vi "TLB Native Dynamic Events ver 0.08a.vi"() -> ()   [LabVIEW 2018]
uses:
  Labview Training Phase 2/Enum Controls/States for Action Engine.ctl
  Type def/TLB event states.ctl
  Type def/TLB MHL States.ctl
  <vilib>/Studica/Studica Toolkit/Background/I2C Channel.ctl
  <vilib>/Studica/Studica Toolkit/NavX/NavX.lvlib
  <vilib>/myRIO/Common/Instrument Driver Framework/myRIO v1.0/AI/typedefs/AI Channels Enum.ctl
  <vilib>/myRIO/Common/Instrument Driver Framework/myRIO v1.0/AI/typedefs/AI Channels List.ctl
  Type def/Type def.ctl
  <vilib>/Studica/Studica Blackhawk/Blackhawk.lvlib
  <vilib>/Studica/Studica Toolkit/Background/Mxp Selection.ctl
  <vilib>/Studica/Studica Toolkit/Background/DIO Channel.ctl
  <vilib>/NI_Real-Time Target Support.lvlib
  <vilib>/ptbypt/NI_PtbyPt.lvlib
  <vilib>/addons/control/pid/NI_PID_pid.lvlib
  Underlying VI's/Webcam FGV Low level ver/State control.ctl
  <vilib>/userdefined/High Color/IMAQdx.ctl
  <vilib>/addons/control/pid/pid.llb/PID (DBL).vi
panel:
  out "Decision":i8
  out "Manual Zero Yaw":bool
  out "Displacement":T1
  out "Fused Heading":dbl
  in  "error in (no error)":errorcluster
  in  "RED LED State":enum16{"OFF", "ON", "BLINK"}(ring)
  in  "GREEN LED State":enum16{"OFF", "ON", "BLINK"}(ring)
  in  "Red LED":bool
  in  "Green LED":bool
  in  "NavX Zero Yaw":bool
  out "Input state":i8
  out "Waveform Chart 2":dbl(graph)
  out "Waveform Chart":dbl(graph)
  in  "STOP":bool
  out "DIO 0":bool
  out "DIO 1":bool
  out "Limit Switch Array":bool[](array[boolean])
  out "error out":errorcluster
  out "L/R average":fxp<+,64,64>
  out "Right Ultrasonic":fxp<+,64,16>
  out "Left Ultrasonic":fxp<+,64,16>
  out "Right IR Sensor":dbl
  out "Left IR Sensor":dbl
  out "Object detection count":T2
  out "Camera error":errorcluster
  in  "Servo Angle":u8(slide) scale=0.0..180.0
  in  "On/Off":bool
  out "Error":errorcluster
  out "element":T3
  out "Action Queue Items":i32
  out "State Logic Queue Items":i32
  out "Action Queues items":string[](array[string])=["Hardware reset", "Software reset", ""]
  out "State logic":T4=enum."Task 2"
  out "Action State":string
  out "Yaw":dbl
  # "TLB FRAMEWORK STATUS"
  # "Camera Status Loop"
  # "Test Programme written by Calvin Loke    Dated: 28 Aug 2019\nTest Programme revised by Dr Alex See   Dated 30 Aug 2019\n\nProgramme version:   TLB Native Dynamic Events ver 0.04b.vi"
  # "Problems now:\nYaw does not work when code is in last state mode\nSlow acceleration due to loop rate?"
  # "Motor Control Loop"
  # "NAVX Control Loop"
  # "Blackhawk status"
  # "Sensor data"
  # "System Health Status Update"
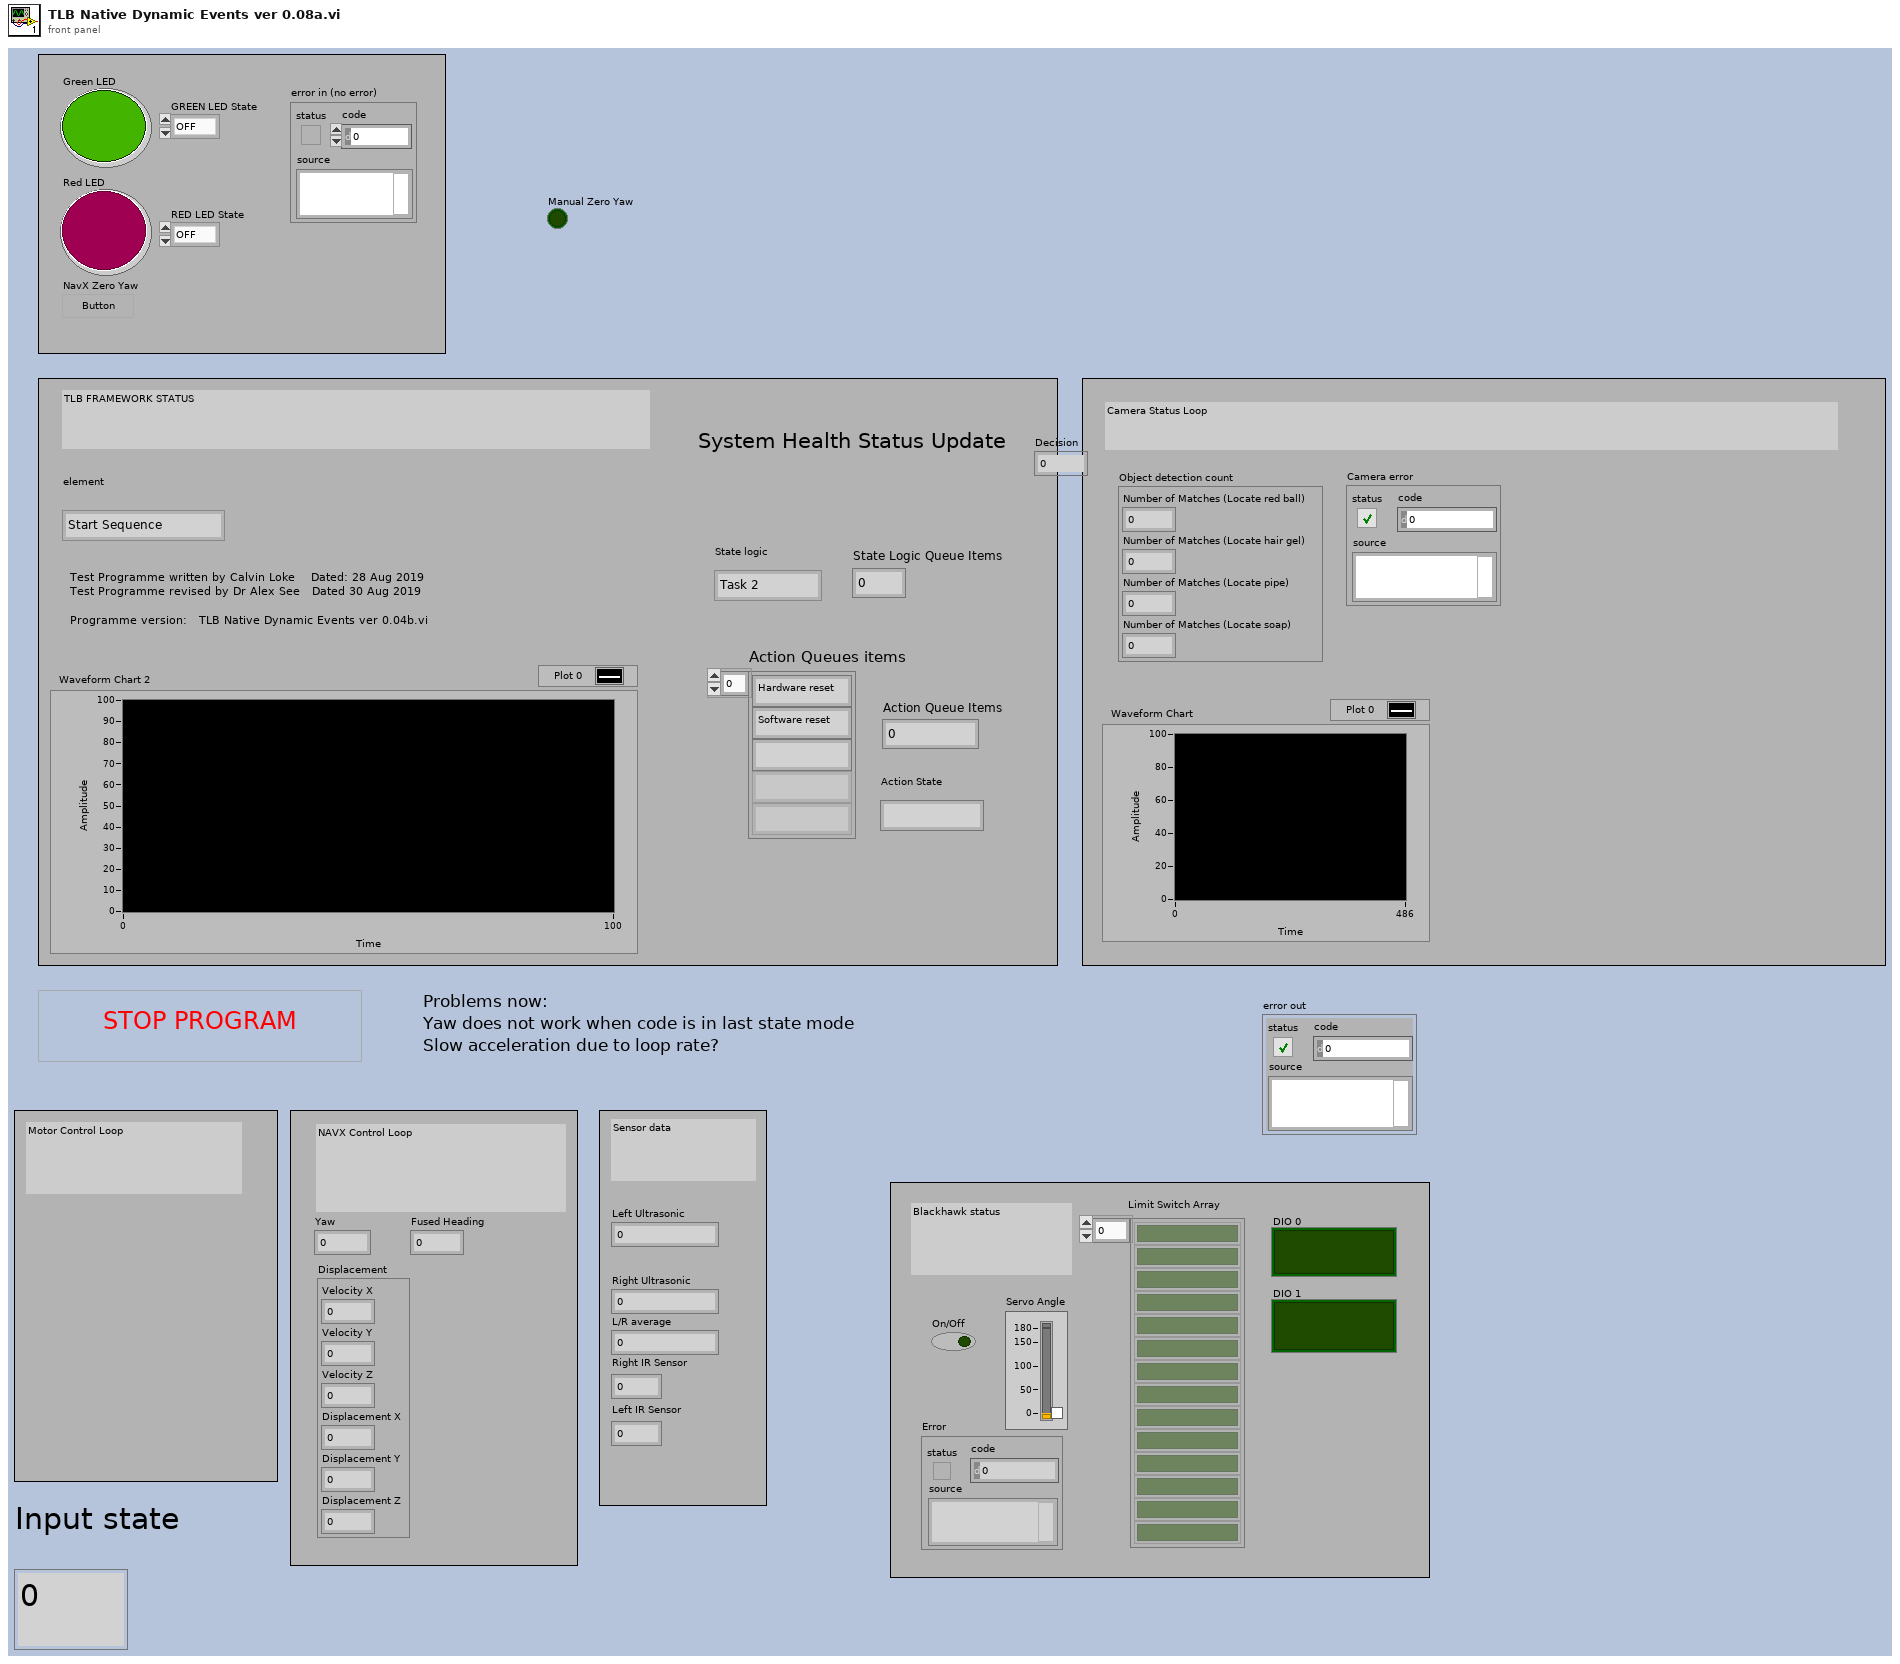
[diagram p1: front panel]
types:
  T1 = cluster{"Velocity X":dbl, "Velocity Y":dbl, "Velocity Z":dbl, "Displacement X":dbl, "Displacement Y":dbl, "Displacement Z":dbl}
  T2 = cluster{"Number of Matches (Locate red ball)":i32, "Number of Matches (Locate hair gel)":i32, "Number of Matches (Locate pipe)":i32, "Number of Matches (Locate soap)":i32}
  T3 = typedef "TLB event states.ctl" = enum16{"Start Sequence", "Exit", "Start Task 1", "Start Task 2", "Start Task 3", "Start Task 4", "Camera vision", "Wall follow mode", "Idle", "Start Drive Straight"}
  T4 = typedef "TLB MHL States.ctl" = enum16{"None", "Startup", "Idle", "Processing", "Shutdown", "Reset", "Task 1", "Task 2", "Task 3", "Task 4", "Task 4a", "Task 4b", "Task 4c", "Task 4d", "Task 4e", "Task 4f", "Task 4g", "Task 4h", "Acquire image", "Wall follow mode", "Autodrive", "Autodrive a"}
  T5 = typedef "States for Action Engine.ctl" = enum16{"Initialize", "Write", "Read"}
  T6 = typedef "DIO Channel.ctl" = enum16{"Not Connected", "A/DIO1", "A/DIO2", "A/DIO3", "A/DIO4", "A/DIO5", "A/DIO6", "A/DIO7", "A/DIO13", "B/DIO1", "B/DIO2", "B/DIO3", "B/DIO4", "B/DIO5", "B/DIO6", "B/DIO7", "B/DIO13", "C/DIO0", "C/DIO1", "C/DIO2", "C/DIO3", "C/DIO4", "C/DIO5", "C/DIO6", "C/DIO7"}
  T7 = typedef "Type def.ctl" = cluster{"Front Ultrasonic Obstruct":bool, "Left Ultrasonic Obstruct":bool, "Right Ultrasonic Obstruct ":bool}
  T8 = typedef "I2C Channel.ctl" = enum16{"Not Connected", "A", "B"}
  T9 = enum16{"LAST STATE", "STOP", "FORWARD", "BACKWARD", "LEFT", "RIGHT", "RCW", "ACW", "INIT", "RESET ENCODERS"}
  T10 = cluster{"proportional gain (Kc)":dbl, "integral time (Ti, min)":dbl, "derivative time (Td, min)":dbl}
  T11 = typedef "State control.ctl" = enum16{"Initialise", "Start camera", "Continuous Acquisition ", "Stop camera", "Dispose all"}
  T12 = typedef "IMAQdx.ctl" = refnum<k21>
  T13 = typedef "Mxp Selection.ctl" = enum16{"MXP A", "MXP B"}
  T14 = enum16{"DISTANCE READ", "STOP", "FORWARD", "BACKWARD", "LEFT", "RIGHT", "RCW", "ACW", "INIT", "RESET ENCODERS"}
  T15 = typedef "AI Channels List.ctl" = T16[]
  T16 = typedef "AI Channels Enum.ctl" = enum16{"Not Connected", "AudioIn/Left", "AudioIn/Right", "C/AI0", "C/AI1", "A/AI0", "A/AI1", "A/AI2", "A/AI3", "A/AI4", "A/AI5", "A/AI6", "A/AI7", "B/AI0", "B/AI1", "B/AI2", "B/AI3", "B/AI4", "B/AI5", "B/AI6", "B/AI7", "AI/AI0", "AI/AI1", "AI/AI2", "AI/AI3", "A/AI0 (DIFF)", "A/AI1 (DIFF)", "A/AI2 (DIFF)", "A/AI3 (DIFF)", "B/AI0 (DIFF)", "B/AI1 (DIFF)", "B/AI2 (DIFF)", "B/AI3 (DIFF)"}
  T17 = cluster{"DIO Channel":T6, "FPGA VI Reference Out":refnum<k20>}
  T18 = typedef "Analog Scaling Constants List.ctl" = T19[]
  T19 = typedef "Analog Scaling Constants.ctl" = cluster{"LSB Weight (Volts)":dbl, "Offset (Volts)":dbl, "Signed?":bool}
  T20 = cluster{"Scale Constants Array":T18, "FPGA Reference Out":refnum<k20>, "AI Channel":T15}
  T21 = cluster{"I2C Channel":T8, "FPGA VI Reference Out":refnum<k20>}
  T22 = typedef "NI_Real-Time Target Support.lvlib/RT CPU Load.ctl" = cluster{"Total (%)":dbl, "Time Critical (%)":dbl, "Timed Structures (%)":dbl, "High (%)":dbl, "Above Normal (%)":dbl, "Normal (%)":dbl, "Background (%)":dbl, "Idle (%)":dbl, "ISR (%)":dbl}
  T23 = cluster{"CPU loads[0]":T22, "CPU loads[1]":T22, "CPU loads[2]":T22, "CPU loads[3]":T22, "CPU loads[4]":T22, "CPU loads[5]":T22, "CPU loads[6]":T22, "CPU loads[7]":T22, "CPU loads[8]":T22}
  T24 = cluster{"I2C Ref Out":cluster{"I2C Channel":T8, "FPGA VI Reference Out":refnum<k20>}, "Connected":bool, "Slave Address (7-bit)":u8, "Registry":u8[]}
  T25 = cluster{"Yaw":dbl, "Roll":dbl, "Pitch":dbl, "Heading":dbl, "Fused Heading":dbl}
  T26 = typedef "IMAQ Image.ctl" = refnum<image>
  T27 = cluster{cluster{"xSpeed":dbl, "ySpeed":dbl, "wSpeed":dbl}, cluster{"xDistance":dbl, "yDistance":dbl, "wDistance":dbl}}
  T28 = cluster{"xDistance":dbl, "yDistance":dbl, "wDistance":dbl}
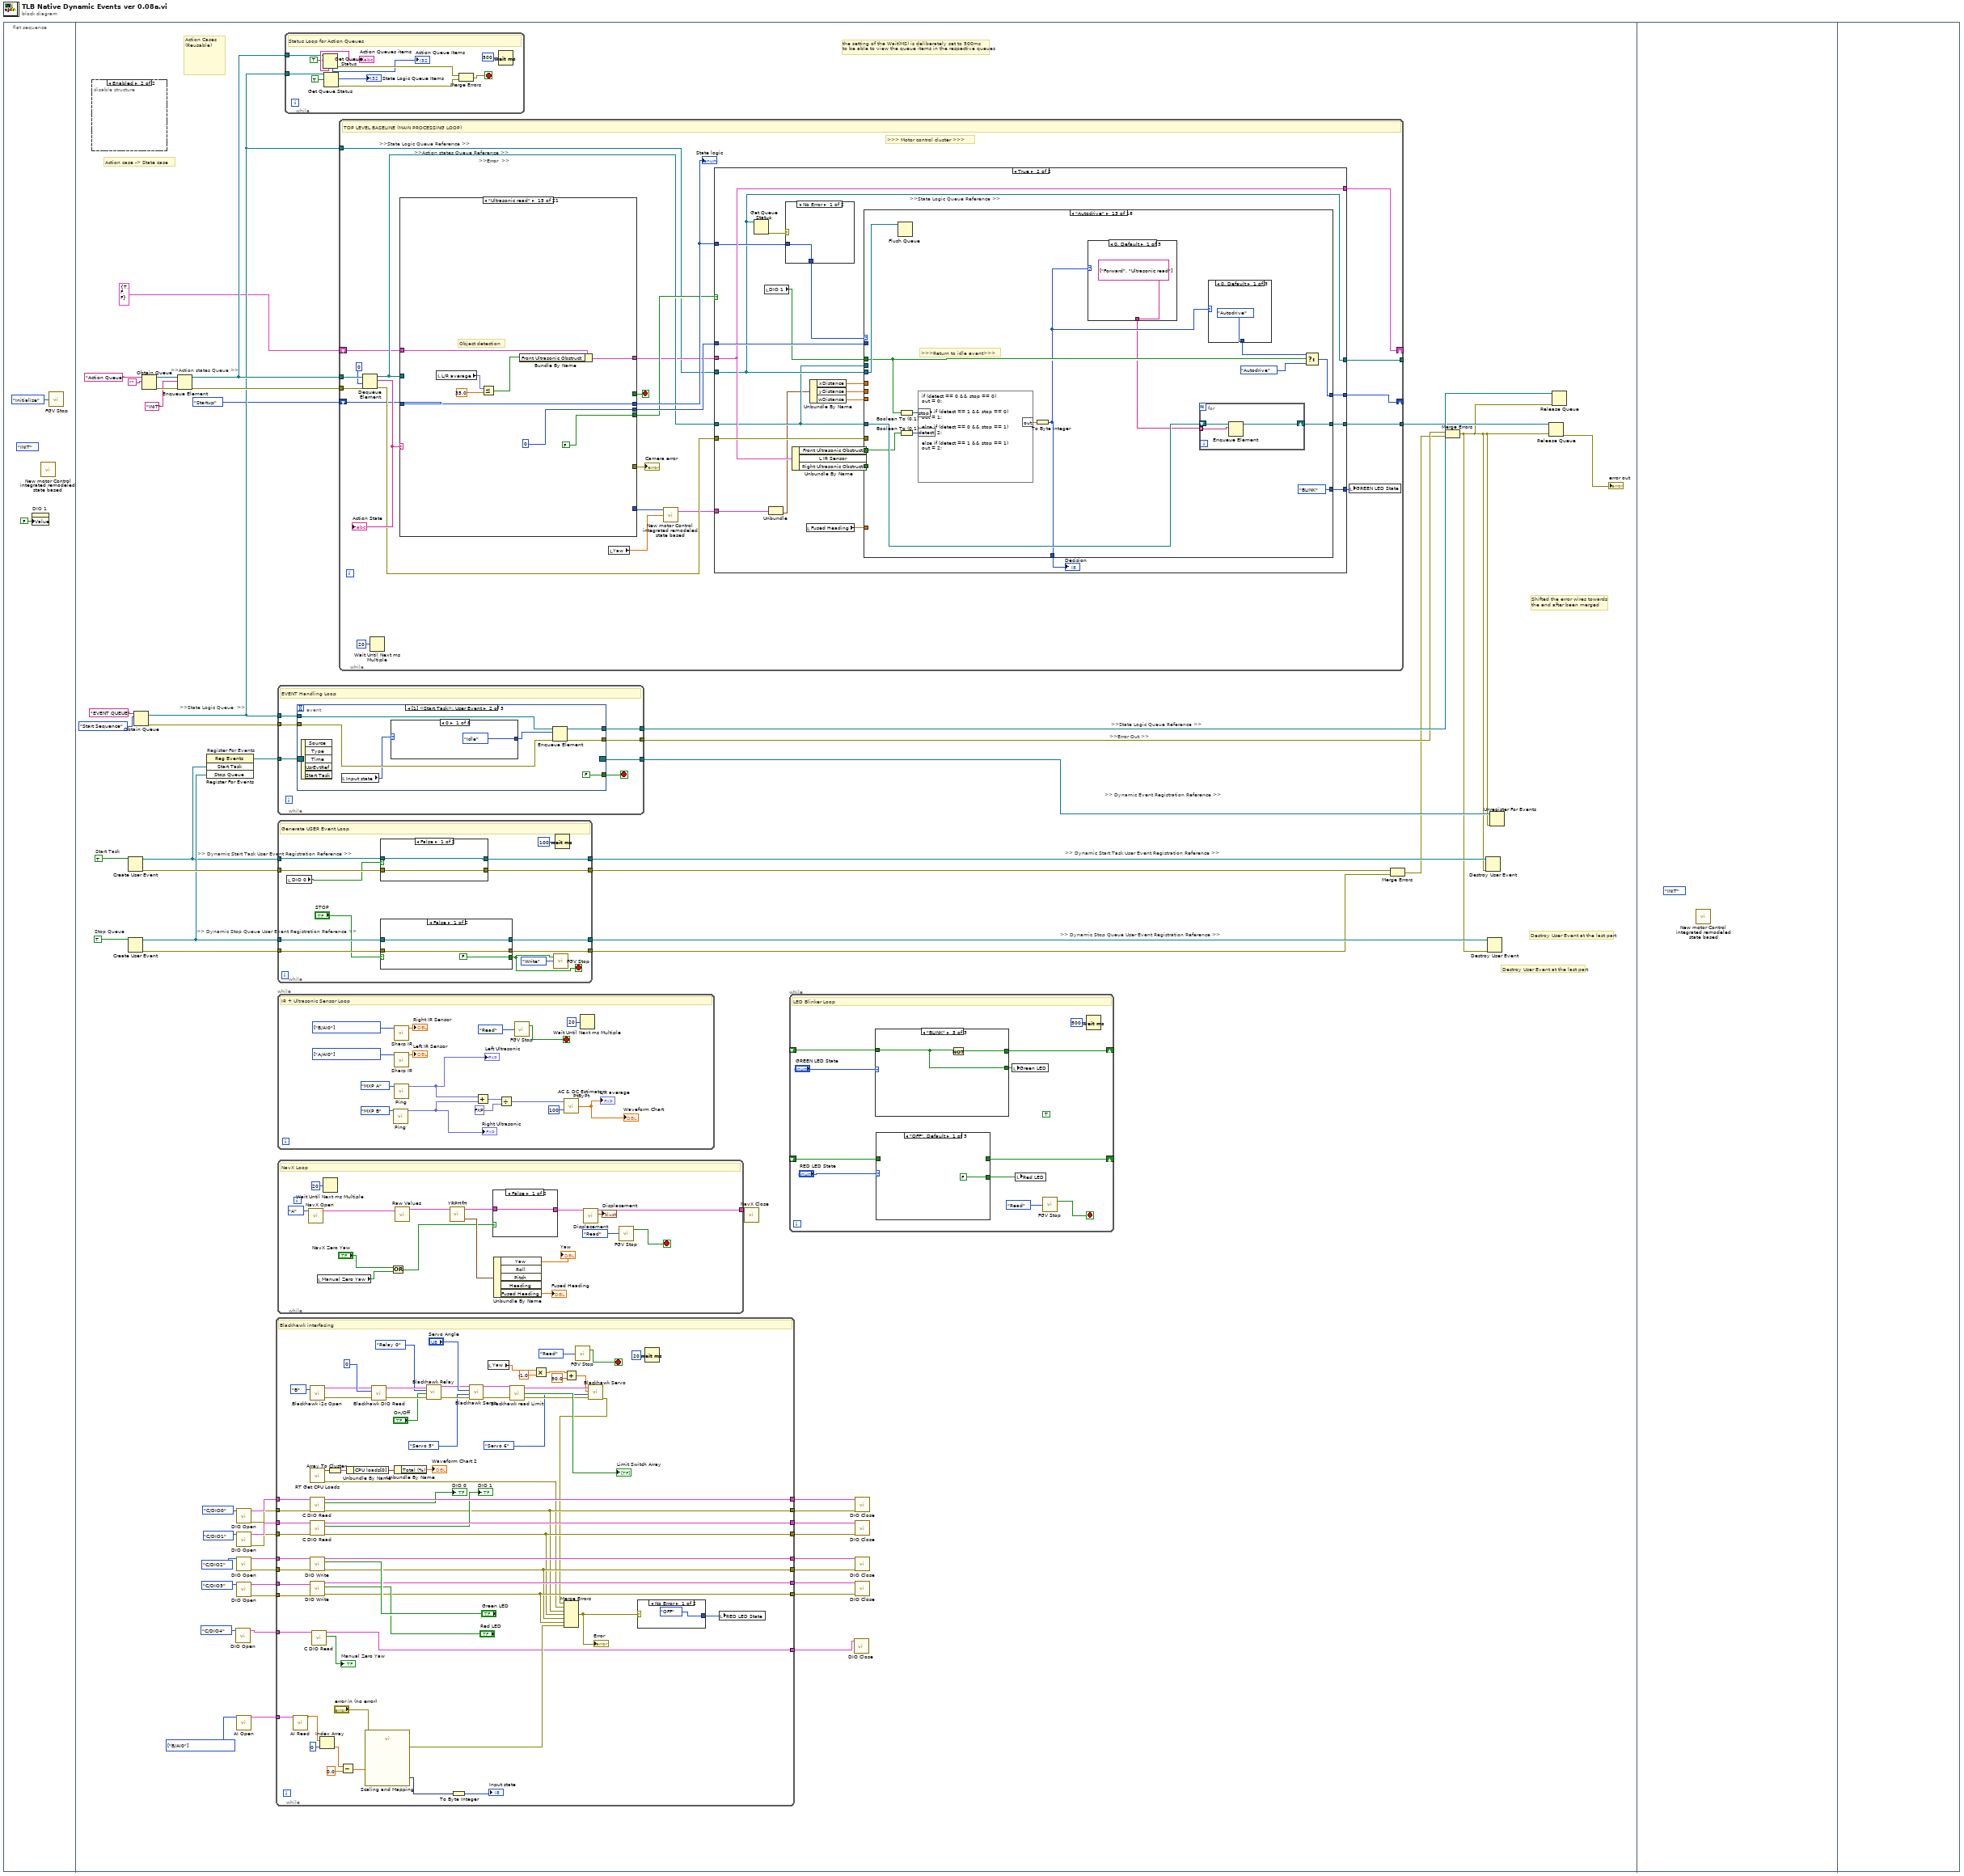
[diagram p0: block diagram]
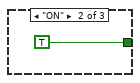
[diagram p2: hidden frame]
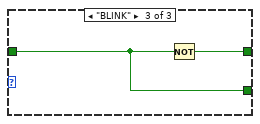
[diagram p3: hidden frame]
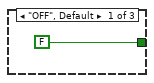
[diagram p4: hidden frame]
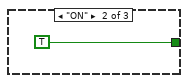
[diagram p5: hidden frame]
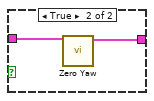
[diagram p6: hidden frame]
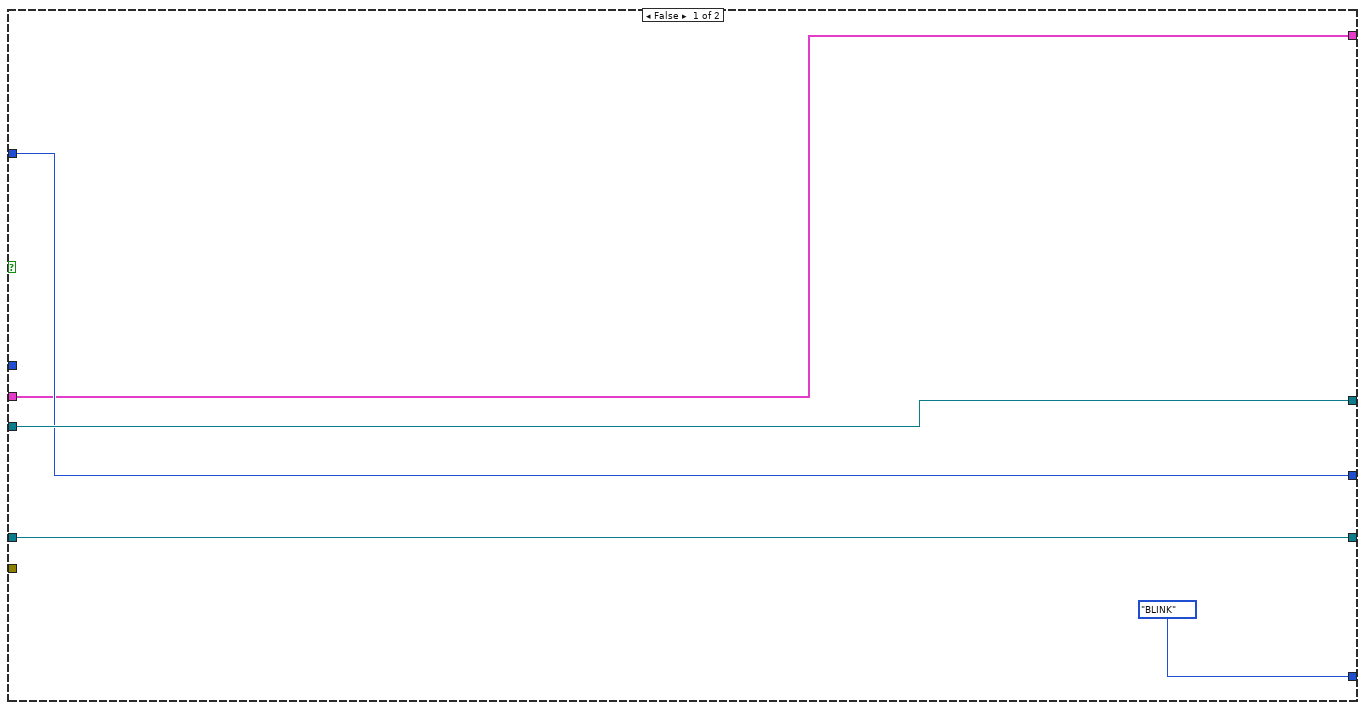
[diagram p7: hidden frame]
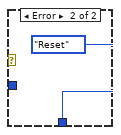
[diagram p8: hidden frame]
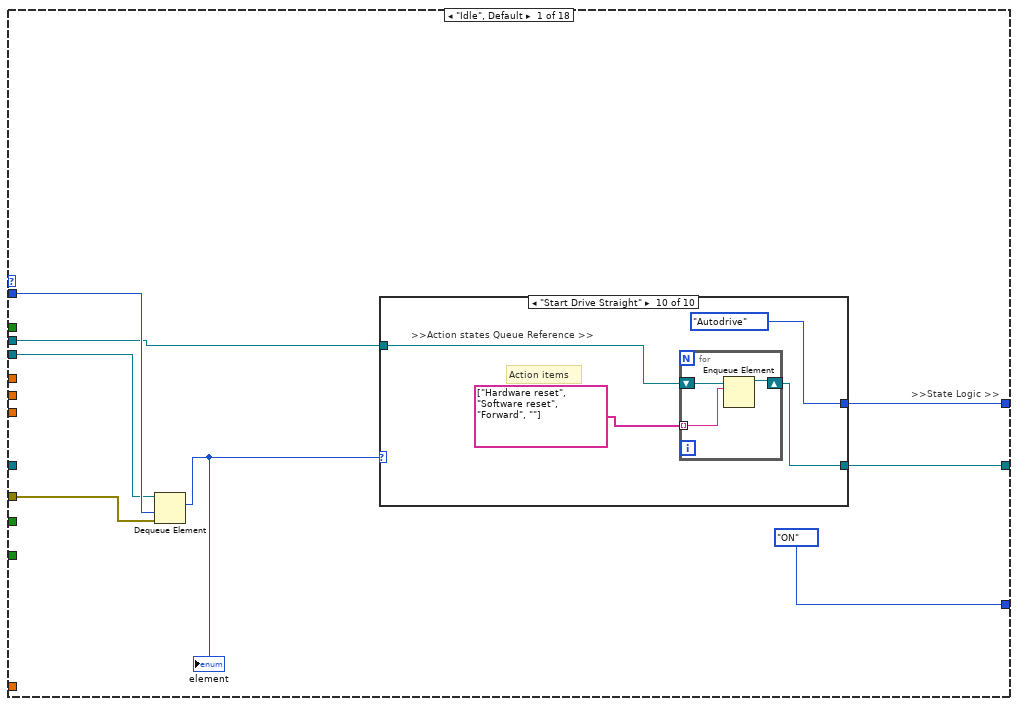
[diagram p9: hidden frame]
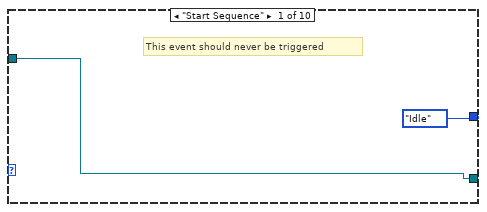
[diagram p10: hidden frame]
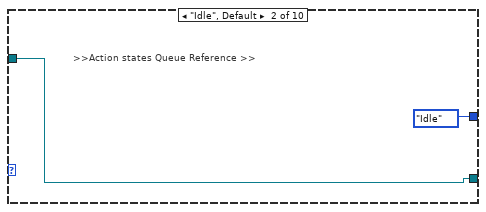
[diagram p11: hidden frame]
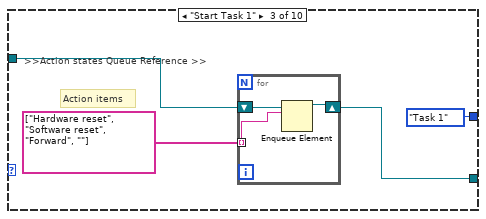
[diagram p12: hidden frame]
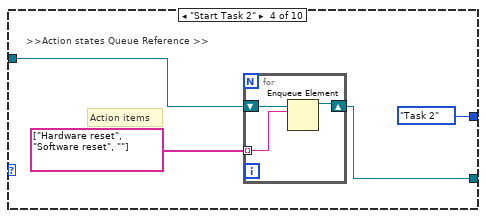
[diagram p13: hidden frame]
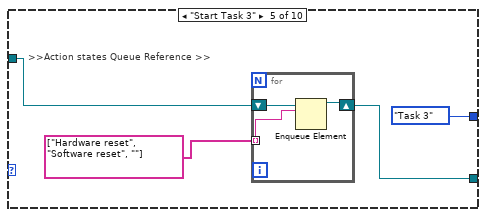
[diagram p14: hidden frame]
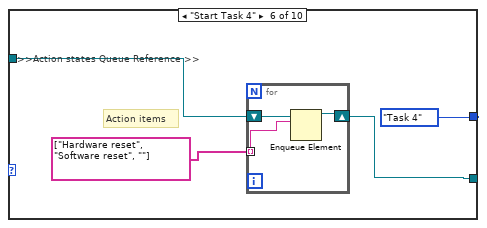
[diagram p15: hidden frame]
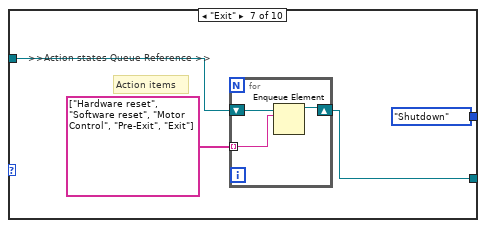
[diagram p16: hidden frame]
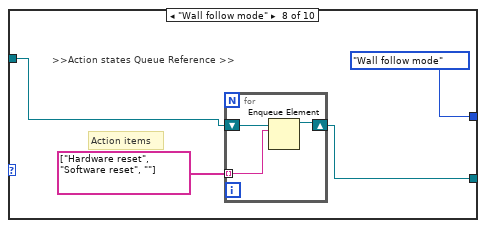
[diagram p17: hidden frame]
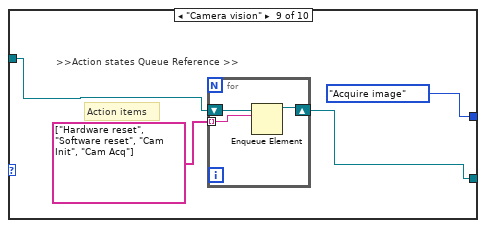
[diagram p18: hidden frame]
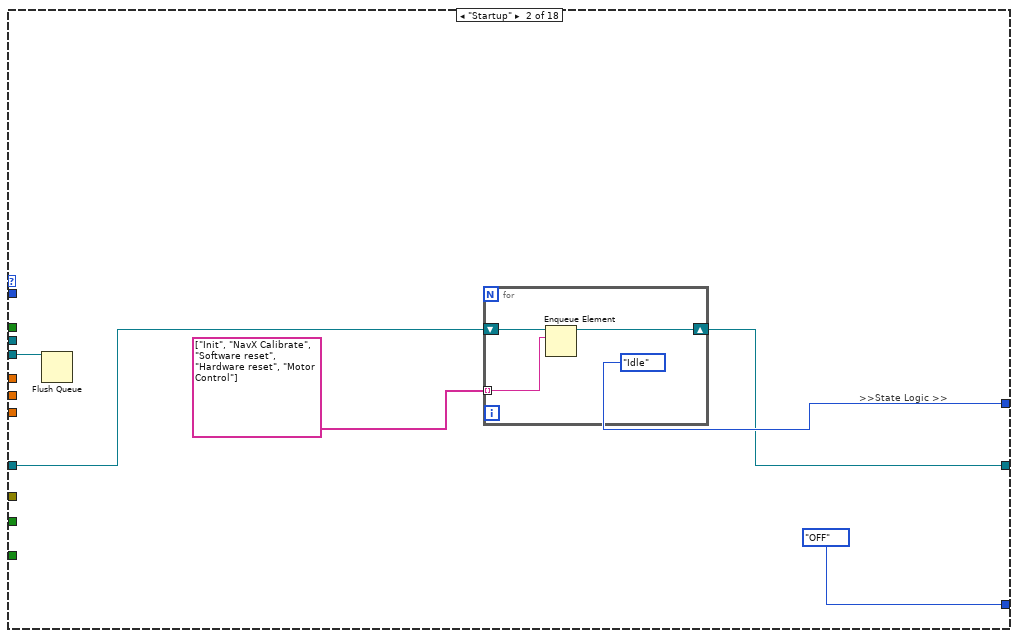
[diagram p19: hidden frame]
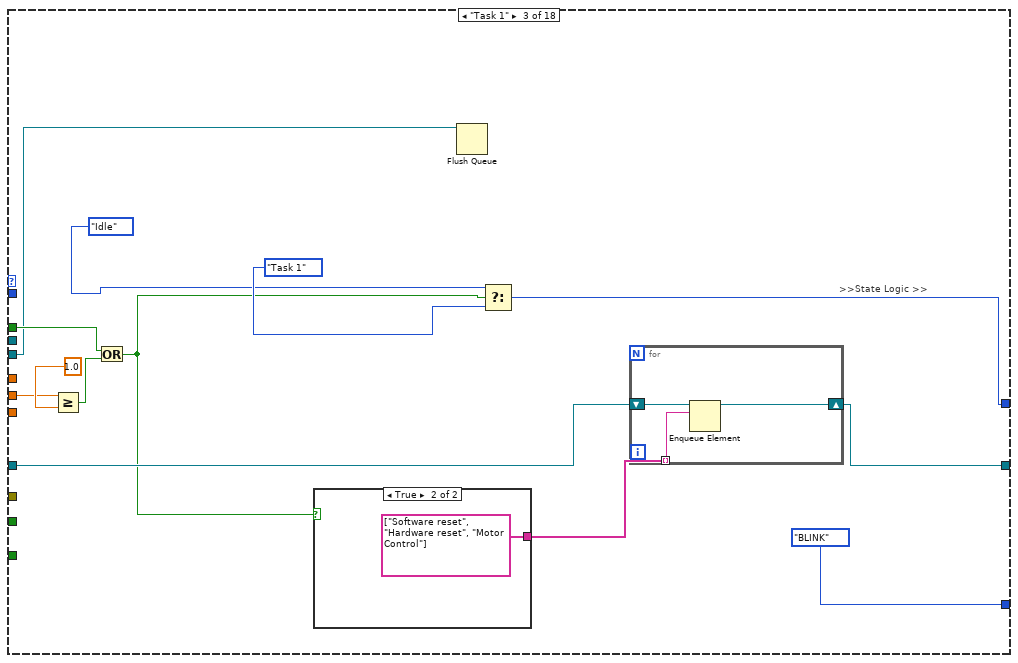
[diagram p20: hidden frame]
diagram:
  n1 = flat-sequence {
    frame #0 {
      (unwired) T14."INIT" ("States")
      n2 = property on="DIO 1" class="Bool (strict)"("Value"=FALSE ("DIO 1")) -> ()  [unwired: 2 in, 2 out]
      n3 = call "New motor Control integrated remodeled state based.vi"() -> ()  [unwired: 3 in, 2 out]
      n4 = call "FGV Stop.vi"("Init/Read/Write State"=States_for_Action_Engine."Initialize") -> ()  [unwired: 2 in, 2 out]
    }
    frame #1 {
      w11 = T15 [enum."B/AI0"] items=["Not Connected", "AudioIn/Left", "AudioIn/Right", "C/AI0", "C/AI1", "A/AI0", "A/AI1", "A/AI2", "A/AI3", "A/AI4", "A/AI5", "A/AI6", "A/AI7", "B/AI0", "B/AI1", "B/AI2", "B/AI3", "B/AI4", "B/AI5", "B/AI6", "B/AI7", "AI/AI0", "AI/AI1", "AI/AI2", "AI/AI3", "A/AI0 (DIFF)", "A/AI1 (DIFF)", "A/AI2 (DIFF)", "A/AI3 (DIFF)", "B/AI0 (DIFF)", "B/AI1 (DIFF)", "B/AI2 (DIFF)", "B/AI3 (DIFF)"] ("AI Channel")
      w59 = TRUE  # Stop Queue
      w58 = TRUE  # Start Task
      # "Action case -> State case"
      # "the setting of the Wait(MS) is deliberately set to 500ms\nto be able to view the queue items in the respective queues"
      # "Action Cases\n(Reusable)"
      # ">>Error Out >>"
      # ">> Dynamic Stop Queue User Event Registration Reference >>"
      # ">> Dynamic Start Task User Event Registration Reference >>"
      # ">> Dynamic Stop Queue User Event Registration Reference >>"
      # ">> Dynamic Start Task User Event Registration Reference >>"
      # ">> Dynamic Event Registration Reference >>"
      # ">>Action states Queue >>"
      # ">>State Logic Queue  >>"
      # ">>State Logic Queue Reference >>"
      # "Destroy User Event at the last part"
      # "Destroy User Event at the last part"
      # "Shifted the error wires towards\nthe end after been merged"
      n5 = disable-structure shown="Enabled" {
        frame Disabled {
          (unwired) variant
          (unwired) TRUE
          n6 = Variant To Data(type="") -> ()  [unwired: 2 in, 2 out]
        }
        frame Enabled {
        }
      }
      n7 = Create User Event(user event datatype=w58) -> (user event=w50:refnum<user-event>, error out=w55:errorcluster)  [unwired: 1 in]
      n8 = Create User Event(user event datatype=w59) -> (user event=w51:refnum<user-event>, error out=w54:errorcluster)  [unwired: 1 in]
      n9 = Obtain Queue(name (unnamed)="EVENT QUEUE", element data type=TLB_event_states."Start Sequence" ("Enum")) -> (queue out=w35:refnum<queue>, error out=w41:errorcluster)  [unwired: 3 in, 1 out]
      n10 = Obtain Queue(name (unnamed)="Action Queue", element data type="") -> (queue out=w44:refnum<queue>, error out=w40:errorcluster)  [unwired: 3 in, 1 out]
      n11 = Enqueue Element(queue=w44, element="INIT", error in (no error)=w40) -> (queue out=w36:refnum<queue>, error out=w39:errorcluster)  [unwired: 1 in, 1 out]
      n12 = register-events "Register For Events"(w50, w51) -> (reference out=w49:refnum<event-registration>)  [unwired: 2 in, 1 out]
      n13 = call <vilib>:"DIO Open.vi"("DIO Channel"=DIO_Channel."C/DIO4") -> ("DIO Info Out"=w5:T17)  [unwired: 9 in, 1 out]
      n14 = call <vilib>:"DIO Open.vi"("DIO Channel"=DIO_Channel."C/DIO0") -> ("error out"=w21:errorcluster, "DIO Info Out"=w27:T17)  [unwired: 9 in]
      n15 = call <vilib>:"DIO Open.vi"("DIO Channel"=DIO_Channel."C/DIO1") -> ("error out"=w19:errorcluster, "DIO Info Out"=w23:T17)  [unwired: 9 in]
      n16 = call <vilib>:"DIO Open.vi"("DIO Channel"=DIO_Channel."C/DIO2") -> ("error out"=w9:errorcluster, "DIO Info Out"=w15:T17)  [unwired: 9 in]
      n17 = call <vilib>:"DIO Open.vi"("DIO Channel"=DIO_Channel."C/DIO3") -> ("error out"=w7:errorcluster, "DIO Info Out"=w14:T17)  [unwired: 9 in]
      n18 = call <vilib>:"AI Open.vi"("AI Channel"=w11) -> ("Analog Info"=w10:T20)  [unwired: 9 in, 1 out]
      n19 = while {
        tunnel: w27 -> [w736]
        tunnel: [w735] -> w26
        tunnel: w23 -> [w734]
        tunnel: [w733] -> w22
        tunnel: w21 -> [w732]
        tunnel: [w701] -> w20
        tunnel: w19 -> [w731]
        tunnel: [w702] -> w18
        tunnel: w15 -> [w725]
        tunnel: w14 -> [w724]
        tunnel: [w721] -> w13
        tunnel: [w720] -> w12
        tunnel: w10 -> [w719]
        tunnel: w9 -> [w712]
        tunnel: [w703] -> w8
        tunnel: w7 -> [w711]
        tunnel: [w704] -> w6
        tunnel: w5 -> [w692]
        tunnel: [w691] -> w3
        stop <- w749 stop-if-true
        # "Blackhawk interfacing"
        n20 = call <vilib>:"AI Read.vi"("Analog Info"=w719) -> ("Array"=w715:dbl[])  [unwired: 9 in, 1 out]
        n21 = call <vilib>:"Blackhawk i2c Open.vi"("I2C Channel"=I2C_Channel."B") -> ("I2C Ref Out"=w727:T21, "error out"=w726:errorcluster)  [unwired: 2 in]
        n22 = call <vilib>:"RT Get CPU Loads.vi"() -> ("error out"=w700:errorcluster, "CPU loads"=w706:T22[])  [unwired: 10 in]
        n23 = call <vilib>:"C DIO Read.vi"("error in (no error)"=w732, "DIO Info In in"=w736) -> ("error out"=w701:errorcluster, "IN"=→"DIO 0":bool, "DIO Info In out"=w735:T17)  [unwired: 7 in]
        n24 = call <vilib>:"C DIO Read.vi"("error in (no error)"=w731, "DIO Info In in"=w734) -> ("error out"=w702:errorcluster, "IN"=→"DIO 1":bool, "DIO Info In out"=w733:T17)  [unwired: 7 in]
        n25 = call <vilib>:"DIO Write.vi"("error in (no error)"=w712, "Input"="Green LED", "DIO Info In"=w725) -> ("error out"=w703:errorcluster, "DIO Info Out"=w721:T17)  [unwired: 7 in]
        n26 = call <vilib>:"DIO Write.vi"("error in (no error)"=w711, "Input"="Red LED", "DIO Info In"=w724) -> ("error out"=w704:errorcluster, "DIO Info Out"=w720:T17)  [unwired: 7 in]
        n27 = call <vilib>:"C DIO Read.vi"("DIO Info In in"=w692) -> ("IN"=→"Manual Zero Yaw":bool, "DIO Info In out"=w691:T17)  [unwired: 8 in, 1 out]
        n28 = Index Array(array=w715, index=0) -> (element=w717:dbl)
        n29 = Array To Cluster(array=w706) -> (cluster=w707:T23)
        n30 = Subtract(x=w717, y=0.0) -> (x-y=w718:dbl)
        n31 = Unbundle By Name(w707) -> ("CPU loads[0]"=w708:T22)
        n32 = call "Scaling and Mapping"("error in (no error)"="error in (no error)", "Signals"=w718) -> ("error out"=w705:errorcluster, "Scaled Signals"=w713:dynamicdata)  [unwired: 8 in]
        n33 = call <vilib>:"Blackhawk DIO Read.vi"("I2C Ref In"=w727, "PIN"=u8 0, "error in (no error)"=w726) -> ("I2C Ref Out"=w747:T21, "error out"=w748:errorcluster)  [unwired: 3 in, 1 out]
        n34 = Unbundle By Name(w708) -> ("Total (%)"=→"Waveform Chart 2":dbl)
        n35 = call <vilib>:"Blackhawk Relay.vi"("error in (no error)"=w748, "On/Off"="On/Off", "Relay"=enum8{"Relay 0", "Relay 1", "Relay 2"}."Relay 0", "I2C Ref In"=w747) -> ("error out"=w744:errorcluster, "I2C Ref Out"=w741:T21)  [unwired: 6 in]
        n36 = To Byte Integer(number=w713) -> (8bit integer=→"Input state":i8)
        n37 = call <vilib>:"Blackhawk Servo.vi"("error in (no error)"=w744, "Servo Select"=enum16{"Servo 5", "Servo 6"}."Servo 5", "Servo Angle"="Servo Angle", "I2C Ref In"=w741) -> ("error out"=w739:errorcluster, "I2C Ref Out"=w738:T21)  [unwired: 6 in]
        n38 = local read "Yaw"() -> (w686:dbl)
        n39 = call <vilib>:"Blackhawk read Limit.vi"("error in (no error)"=w739, "I2C Ref In"=w738) -> ("error out"=w696:errorcluster, "Limit Switch Array"=→"Limit Switch Array":bool[], "I2C Ref Out"=w694:T21)  [unwired: 1 in]
        n40 = Multiply(x=w686, y=-1.0) -> (x*y=w687:dbl)
        n41 = Add(x=w687, y=90.0) -> (x+y=w688:dbl)
        n42 = call "FGV Stop.vi"("Init/Read/Write State"=States_for_Action_Engine."Read") -> ("Output node"=w749:bool)  [unwired: 2 in, 1 out]
        n43 = call <vilib>:"Blackhawk Servo.vi"("error in (no error)"=w696, "Servo Select"=enum16{"Servo 5", "Servo 6"}."Servo 6", "Servo Angle"=w688, "I2C Ref In"=w694) -> ("error out"=w695:errorcluster)  [unwired: 6 in, 1 out]
        n44 = Merge Errors(w695, w700, w701, w702, w703, w704, w705) -> (w699:errorcluster)
        "Error" <- w699
        n45 = case shown="No Error" w699 {
          tunnel: [enum16{"OFF", "ON", "BLINK"}."OFF" ("RED LED State") enum16{"OFF", "ON", "BLINK"}."BLINK" ("RED LED State")] -> w710
          frame No Error {
          }
          frame Error {
          }
        }
        n46 = Wait (ms)(milliseconds to wait=u32 20) -> ()  [unwired: 1 out]
        n47 = local write "RED LED State"(w710) -> ()
      }
      n48 = while {
        tunnel: w49 -> [w629]
        tunnel: [w628] -> w48
        tunnel: w35 -> [w626]
        tunnel: [w625] -> w47
        tunnel: w41 -> [w624]
        tunnel: [w623] -> w38
        stop <- w627 stop-if-true
        # "EVENT Handling Loop"
        n49 = event shown="[1] <Start Task>: User Event" {
          selector: w629 -> [_ _ _]
          dyn-events: [_ _ _] -> w628
          timeout: _ -> [_ _ _]
          tunnel: [FALSE FALSE w656] -> w627
          tunnel: w626 -> [w634 w641 w654]
          tunnel: [w633 w640 w655] -> w625
          tunnel: w624 -> [w631 w639 w652]
          tunnel: [w630 w638 w651] -> w623
          event Timeout {
            n50 = event-data() -> ()  [unwired: 1 in, 3 out]
            n51 = Enqueue Element(queue=w634, element=TLB_event_states."Idle" ("Enum"), error in (no error)=w631) -> (queue out=w633:refnum<queue>, error out=w630:errorcluster)  [unwired: 1 in, 1 out]
          }
          event User Event {
            n52 = event-data() -> ()  [unwired: 1 in, 5 out]
            n53 = local read "Input state"() -> (w637:i8)
            n54 = case shown="0" w637 {
              tunnel: [TLB_event_states."Idle" ("Enum") TLB_event_states."Start Task 1" ("Enum") TLB_event_states."Start Task 2" ("Enum") TLB_event_states."Start Task 3" ("Enum") TLB_event_states."Start Task 4" ("Enum") TLB_event_states."Wall follow mode" ("Enum") TLB_event_states."Camera vision" ("Enum") TLB_event_states."Start Drive Straight" ("Enum")] -> w636
              frame 0 {
              }
              frame 1 {
              }
              frame 2 {
              }
              frame 3, Default {
              }
              frame 4 {
              }
              frame 5 {
              }
              frame 6 {
              }
              frame 7 {
              }
            }
            n55 = Enqueue Element(queue=w641, element=w636, error in (no error)=w639) -> (queue out=w640:refnum<queue>, error out=w638:errorcluster)  [unwired: 1 in, 1 out]
          }
          event User Event {
            n56 = event-data() -> ("Stop Queue"=w656:bool)  [unwired: 1 in, 4 out]
            n57 = Enqueue Element At Opposite End(queue=w654, element=TLB_event_states."Exit" ("Enum"), error in (no error)=w652) -> (queue out=w655:refnum<queue>, error out=w651:errorcluster)  [unwired: 1 in, 1 out]
          }
        }
      }
      n58 = while {
        tunnel: w50 -> [w668]
        tunnel: w51 -> [w667]
        tunnel: [w666] -> w57
        tunnel: [w665] -> w56
        tunnel: w55 -> [w664]
        tunnel: [w663] -> w53
        tunnel: w54 -> [w662]
        tunnel: [w661] -> w52
        stop <- w659 stop-if-true
        # "Generate USER Event Loop"
        n59 = local read "DIO 0"() -> (w658:bool)
        n60 = case shown="False" w658 {
          selector: w658 -> [_ w680]
          tunnel: w668 -> [w679 w684]
          tunnel: [w679 w683] -> w665
          tunnel: w664 -> [w678 w682]
          tunnel: [w678 w681] -> w663
          frame False {
          }
          frame True {
            n61 = Generate User Event(user event=w684, event data cluster=w680, error in=w682) -> (user event out=w683:refnum<user-event>, error out=w681:errorcluster)  [unwired: 1 in]
          }
        }
        n62 = case shown="False" "STOP" {
          selector: "STOP" -> [_ w673]
          tunnel: w667 -> [w672 w677]
          tunnel: [w672 w676] -> w666
          tunnel: w662 -> [w671 w675]
          tunnel: [w671 w674] -> w661
          tunnel: [FALSE w673] -> w659
          frame False {
          }
          frame True {
            n63 = Generate User Event(user event=w677, event data cluster=w673, error in=w675) -> (user event out=w676:refnum<user-event>, error out=w674:errorcluster)  [unwired: 1 in]
          }
        }
        n64 = call "FGV Stop.vi"("Init/Read/Write State"=States_for_Action_Engine."Write", "Input Node"=w659) -> ()  [unwired: 1 in, 2 out]
        n65 = Wait (ms)(milliseconds to wait=u32 100) -> ()  [unwired: 1 out]
      }
      n66 = while {
        stop <- w605 stop-if-true
        w610 = T15 [enum."A/AI0"] items=["Not Connected", "AudioIn/Left", "AudioIn/Right", "C/AI0", "C/AI1", "A/AI0", "A/AI1", "A/AI2", "A/AI3", "A/AI4", "A/AI5", "A/AI6", "A/AI7", "B/AI0", "B/AI1", "B/AI2", "B/AI3", "B/AI4", "B/AI5", "B/AI6", "B/AI7", "AI/AI0", "AI/AI1", "AI/AI2", "AI/AI3", "A/AI0 (DIFF)", "A/AI1 (DIFF)", "A/AI2 (DIFF)", "A/AI3 (DIFF)", "B/AI0 (DIFF)", "B/AI1 (DIFF)", "B/AI2 (DIFF)", "B/AI3 (DIFF)"] ("AI Channel")
        w611 = T15 [enum."B/AI0"] items=["Not Connected", "AudioIn/Left", "AudioIn/Right", "C/AI0", "C/AI1", "A/AI0", "A/AI1", "A/AI2", "A/AI3", "A/AI4", "A/AI5", "A/AI6", "A/AI7", "B/AI0", "B/AI1", "B/AI2", "B/AI3", "B/AI4", "B/AI5", "B/AI6", "B/AI7", "AI/AI0", "AI/AI1", "AI/AI2", "AI/AI3", "A/AI0 (DIFF)", "A/AI1 (DIFF)", "A/AI2 (DIFF)", "A/AI3 (DIFF)", "B/AI0 (DIFF)", "B/AI1 (DIFF)", "B/AI2 (DIFF)", "B/AI3 (DIFF)"] ("AI Channel")
        # "IR + Ultrasonic Sensor Loop"
        n67 = call <vilib>:"Ping.vi"("Mxp Side"=Mxp_Selection."MXP B") -> ("CM"=w599:fxp<+,64,16>)  [unwired: 8 in, 2 out]
        "Right Ultrasonic" <- w599
        n68 = call <vilib>:"Ping.vi"("Mxp Side"=Mxp_Selection."MXP A") -> ("CM"=w600:fxp<+,64,16>)  [unwired: 8 in, 2 out]
        "Left Ultrasonic" <- w600
        n69 = call <vilib>:"Sharp IR.vi"("AI Channel"=w611) -> ("Sharp IR Distance"=→"Right IR Sensor":dbl)  [unwired: 8 in, 2 out]
        n70 = call <vilib>:"Sharp IR.vi"("AI Channel"=w610) -> ("Sharp IR Distance"=→"Left IR Sensor":dbl)  [unwired: 8 in, 2 out]
        n71 = Add(x=w600, y=w599) -> (x+y=w602:fxp<+,64,17>)
        n72 = Divide(x=w602, y=fxp<+,64,17> 2.0) -> (x/y=w598:fxp<+,64,64>)
        n73 = call "FGV Stop.vi"("Init/Read/Write State"=States_for_Action_Engine."Read") -> ("Output node"=w605:bool)  [unwired: 2 in, 1 out]
        n74 = call <vilib>:"AC & DC Estimator PtByPt.vi"("signal"=w598, "sample length"=100) -> ("DC estimate (V)"=→"L/R average" →"Waveform Chart":dbl)  [unwired: 1 in, 2 out]
        n75 = Wait Until Next ms Multiple(millisecond multiple=u32 20) -> ()  [unwired: 1 out]
      }
      n76 = while {
        tunnel: [w85] -> w28
        stop <- w93 stop-if-true
        # "NavX Loop"
        n77 = call <vilib>:"NavX Open.vi"("I2C Channel"=I2C_Channel."A") -> ("NavX Info"=w87:T24)  [unwired: 9 in, 1 out]
        n78 = local read "Manual Zero Yaw"() -> (w81:bool)
        n79 = Wait Until Next ms Multiple(millisecond multiple=u32 20) -> ()  [unwired: 1 out]
        n80 = Or(x="NavX Zero Yaw", y=w81) -> (x .or. y?=w82:bool)
        n81 = call <vilib>:"Raw Values.vi"("NavX Info In"=w87) -> ("NavX Info Out"=w90:T24)  [unwired: 8 in, 1 out]
        n82 = call <vilib>:"YRPHfH.vi"("NavX Info In"=w90) -> ("YRPHfH"=w91:T25, "NavX Info Out"=w89:T24)  [unwired: 3 in]
        n83 = case shown="False" w82 {
          tunnel: [w95 w97] -> w86
          tunnel: w89 -> [w95 w96]
          frame False {
          }
          frame True {
            n84 = call <vilib>:"Zero Yaw.vi"("NavX Info In"=w96) -> ("NavX Info Out"=w97:T24)  [unwired: 10 in]
          }
        }
        n85 = Unbundle By Name(w91) -> ("Yaw"=→"Yaw":dbl, "Fused Heading"=→"Fused Heading":dbl)  [unwired: 3 out]
        n86 = call <vilib>:"Displacement.vi"("NavX Info In"=w86) -> ("Displacement"=→"Displacement":T1, "NavX Info Out"=w85:T24)  [unwired: 9 in]
        n87 = call "FGV Stop.vi"("Init/Read/Write State"=States_for_Action_Engine."Read") -> ("Output node"=w93:bool)  [unwired: 2 in, 1 out]
      }
      n88 = while {
        tunnel: w36 -> [w620]
        tunnel: w35 -> [w617]
        stop <- w614 stop-if-true
        # "Status Loop for Action Queues"
        n89 = Get Queue Status(queue=w620, return elements? (F)=TRUE) -> (error out=w616:errorcluster, # elements in queue=→"Action Queue Items":i32, elements=→"Action Queues items":string[])  [unwired: 1 in, 5 out]
        n90 = Get Queue Status(queue=w617, return elements? (F)=TRUE) -> (# pending remove=→"State Logic Queue Items":i32, error out=w615:errorcluster)  [unwired: 1 in, 6 out]
        n91 = Merge Errors(w616, w615) -> (w614:errorcluster)
        n92 = Wait (ms)(milliseconds to wait=u32 500) -> ()  [unwired: 1 out]
      }
      n93 = while {
        tunnel: w35 -> [w104]
        shift-right: [w115] -> _
        shift-left: TLB_MHL_States."Startup" ("Enum") -> [w109]
        tunnel: w36 -> [w120]
        tunnel: w39 -> [w118]
        tunnel: [w117] -> _
        tunnel: [w116] -> w31
        shift-right: [w106] -> _
        shift-left: T7 {"Front Ultrasonic Obstruct"=TRUE, "Left Ultrasonic Obstruct"=FALSE, "Right Ultrasonic Obstruct "=FALSE} -> [w108]
        stop <- w102 stop-if-true
        # ">>> Motor control cluster >>>"
        # ">>Error  >>"
        # ">>Action states Queue Reference >>"
        # ">>State Logic Queue Reference >>"
        # "TOP LEVEL BASELINE (MAIN PROCESSING LOOP)"
        n94 = Dequeue Element(queue=w120, timeout in ms (-1)=0, error in (no error)=w118) -> (queue out=w110:refnum<queue>, element=w119:string, error out=w111:errorcluster)  [unwired: 1 out]
        "Action State" <- w119
        n95 = Wait Until Next ms Multiple(millisecond multiple=u32 20) -> ()  [unwired: 1 out]
        n96 = case shown="\"Ultrasonic read\"" w119 {
          tunnel: [w446 w461 w468 w473 w479 w486 w492 w496 w504 w509 w518 w525 TLB_MHL_States."Shutdown" ("Enum") w535 w544 w547 w558 w569 w577 w589 w593] -> w121
          tunnel: [w449 0 0 0 0 0 0 0 0 0 0 0 0 0 0 0 0 0 0 0 0] -> w114
          tunnel: [TRUE FALSE FALSE FALSE FALSE FALSE FALSE FALSE FALSE FALSE FALSE FALSE FALSE FALSE FALSE FALSE FALSE FALSE FALSE FALSE FALSE] -> w113
          tunnel: w110 -> [_ _ _ _ _ _ _ _ _ _ _ _ _ _ _ _ _ _ _ _ _]
          tunnel: w109 -> [w446 w461 w468 w473 w479 w486 w492 w496 w504 w509 w518 w525 _ w535 w544 w547 w558 w569 w577 w589 w593]
          tunnel: w108 -> [w447 w456 w464 w474 w476 w482 w488 w494 w500 w506 w515 w521 w528 w536 w543 w550 w559 w570 w576 w586 w594]
          tunnel: [w447 w455 w463 w474 w476 w482 w488 w494 w500 w506 w514 w521 w528 w536 w540 w549 w559 w570 w576 w586 w594] -> w107
          tunnel: [_ _ _ _ _ _ _ _ _ _ _ _ _ _ _ _ _ w560 w572 w580 _] -> w105
          tunnel: [_ _ _ _ _ _ _ _ _ _ _ _ TRUE _ _ _ _ _ _ _ _] -> w102
          tunnel: [T9."LAST STATE" ("Move mode") T9."INIT" ("Move mode") T9."FORWARD" ("Move mode") T9."LAST STATE" ("Move mode") T9."BACKWARD" ("Move mode") T9."RIGHT" ("Move mode") T9."LEFT" ("Move mode") T9."RCW" ("Move mode") T9."ACW" ("Move mode") T9."STOP" ("Move mode") _ T9."RESET ENCODERS" ("Move mode") T9."INIT" ("Move mode") T9."INIT" ("Move mode") _ _ _ _ _ _ _] -> w100
          frame "No action", Default {
            n97 = case shown="\"Startup\", Default" w446 {
              tunnel: [0 100] -> w449
              frame "Startup", Default {
              }
              frame "Idle" {
              }
            }
            n98 = local write "NavX Zero Yaw"(FALSE ("NavX Zero Yaw")) -> ()
          }
          frame "Init" {
            # ">>State Logic  >>"
            n99 = local write "Servo Angle"(u8 90 ("Servo Angle")) -> ()
            n100 = Bundle By Name(cluster=w456, "Front Ultrasonic Obstruct"=FALSE ("Object detected"), "L IR Sensor"=0.0, "Right Ultrasonic Obstruct"=FALSE ("In move state?")) -> (w455:T7)
          }
          frame "Forward" {
            n101 = local write "NavX Zero Yaw"(FALSE ("NavX Zero Yaw")) -> ()
            n102 = Bundle By Name(cluster=w464, "Right Ultrasonic Obstruct"=TRUE ("In move state?")) -> (w463:T7)
          }
          frame " Motor Control" {
          }
          frame "Reverse" {
            n103 = local write "NavX Zero Yaw"(FALSE ("NavX Zero Yaw")) -> ()
          }
          frame "Right" {
            n104 = local write "NavX Zero Yaw"(FALSE ("NavX Zero Yaw")) -> ()
          }
          frame "Left" {
            n105 = local write "NavX Zero Yaw"(FALSE ("NavX Zero Yaw")) -> ()
          }
          frame "Rotate CW" {
            n106 = local write "NavX Zero Yaw"(FALSE ("NavX Zero Yaw")) -> ()
          }
          frame "Rotate ACW" {
            n107 = local write "NavX Zero Yaw"(FALSE ("NavX Zero Yaw")) -> ()
          }
          frame "Stop" {
            n108 = local write "NavX Zero Yaw"(FALSE ("NavX Zero Yaw")) -> ()
          }
          frame "Software reset" {
            w511 = FALSE ("NavX Zero Yaw")
            n109 = Wait (ms)(milliseconds to wait=u32 20) -> ()  [unwired: 1 out]
            n110 = local write "NavX Zero Yaw"(w511) -> ()
            n111 = Bundle By Name(cluster=w515, "Front Ultrasonic Obstruct"=w511, "L IR Sensor"=0.0, "Right Ultrasonic Obstruct"=w511) -> (w514:T7)
          }
          frame "Hardware reset" {
            n112 = Wait (ms)(milliseconds to wait=u32 100) -> ()  [unwired: 1 out]
            n113 = local write "NavX Zero Yaw"(TRUE ("NavX Zero Yaw")) -> ()
          }
          frame "Exit" {
          }
          frame "Pre-Exit" {
          }
          frame "Ultrasonic read" {
            # "Object detection"
            n114 = local read "L/R average"() -> (w537:fxp<+,64,64>)
            n115 = Less Or Equal?(x=w537, y=35.0) -> (x <= y?=w538:bool)
            n116 = Bundle By Name(cluster=w543, "Front Ultrasonic Obstruct"=w538) -> (w540:T7)
          }
          frame "IR Sensor Read" {
            n117 = local read "Left IR Sensor"() -> (w548:dbl)
            n118 = Bundle By Name(cluster=w550, "L IR Sensor"=w548) -> (w549:T7)
          }
          frame "Calculate" {
            n119 = Unbundle By Name(w559) -> ("L IR Sensor"=w554:dbl)
            n120 = call-poly <vilib>:"PID.vi"("output range"=cluster{"output high":dbl, "output low":dbl} {"output high"=0.3, "output low"=-0.3}, "PID gains"=T10 {"proportional gain (Kc)"=0.01, "integral time (Ti, min)"=0.0, "derivative time (Td, min)"=0.0}, "process variable"=w554, "setpoint"=20.0) -> ("output"=w551:dbl)  [unwired: 6 in, 1 out]
            n121 = Negate(x=w551) -> ()  [unwired: 1 out]
          }
          frame "Cam Init" {
            n122 = call "Low-Level Grab.vi"("States"=State_control."Initialise", "Session In"=T12 "cam1") -> ("error out"=w561:errorcluster, "Session Out"=w562:T12)  [unwired: 7 in, 1 out]
            n123 = call "Low-Level Grab.vi"("error in (no error)"=w561, "States"=State_control."Start camera", "Session In"=w562) -> ("error out"=w560:errorcluster)  [unwired: 6 in, 2 out]
            n124 = local write "Servo Angle"(u8 170 ("Servo Angle")) -> ()
          }
          frame "Cam Acq" {
            n125 = call "Low-Level Grab.vi"("States"=State_control."Continuous Acquisition ") -> ("error out"=w573:errorcluster, "Image Out"=w574:T26)  [unwired: 8 in, 1 out]
            n126 = call "All object detection ver2.vi"("Image In"=w574, "error in"=w573) -> ("Object detection count"=→"Object detection count":T2, "error out"=w572:errorcluster)  [unwired: 1 out]
          }
          frame "Cam Exit" {
            n127 = call "Low-Level Grab.vi"("States"=State_control."Stop camera") -> ("error out"=w581:errorcluster, "Session Out"=w583:T12)  [unwired: 8 in, 1 out]
            n128 = local write "Servo Angle"(u8 90 ("Servo Angle")) -> ()
            n129 = call "Low-Level Grab.vi"("error in (no error)"=w581, "States"=State_control."Dispose all", "Session In"=w583) -> ("error out"=w580:errorcluster)  [unwired: 6 in, 2 out]
          }
          frame "NavX Calibrate" {
            # "Adds a 15 second delay to the startup process \nfor the NavX to calibrate"
            n130 = Wait (ms)(milliseconds to wait=u32 15000) -> ()  [unwired: 1 out]
          }
        }
        "State logic" <- w121
        "Camera error" <- w105
        n131 = local read "Yaw"() -> (w98:dbl)
        n132 = call "New motor Control integrated remodeled state based.vi"("Yaw"=w98, "States"=w100) -> ("Speed and distance cluster"=w99:T27)  [unwired: 1 in, 1 out]
        n133 = case shown="True" w113 {
          tunnel: w121 -> [w125 w136]
          tunnel: w104 -> [w126 w135]
          tunnel: w110 -> [w124 w131]
          tunnel: [w126 w135] -> w117
          tunnel: [w124 w147] -> w116
          tunnel: [w125 w146] -> w115
          tunnel: w111 -> [_ w145]
          tunnel: w114 -> [_ w144]
          tunnel: w107 -> [w123 w138]
          tunnel: [w123 w138] -> w106
          tunnel: [enum16{"OFF", "ON", "BLINK"}."BLINK" ("GREEN LED State") w132] -> w101
          tunnel: w99 -> [_ w129]
          frame False {
          }
          frame True {
            # ">>State Logic Queue Reference >>"
            n134 = Get Queue Status(queue=w135) -> (error out=w134:errorcluster)  [unwired: 2 in, 7 out]
            n135 = local read "DIO 1"() -> (w133:bool)
            n136 = Unbundle(w129) -> (w128:T28)  [unwired: 1 out]
            n137 = case shown="No Error" w134 {
              tunnel: [w148 TLB_MHL_States."Reset" ("Enum")] -> w137
              tunnel: w136 -> [w148 _]
              frame No Error {
              }
              frame Error {
              }
            }
            n138 = Unbundle By Name(w138) -> ("Front Ultrasonic Obstruct"=w139:bool, "Right Ultrasonic Obstruct"=w130:bool)  [unwired: 1 out]
            n139 = local read "Fused Heading"() -> (w140:dbl)
            n140 = Unbundle By Name(w128) -> ("xDistance"=w141:dbl, "yDistance"=w143:dbl, "wDistance"=w142:dbl)
            n141 = case shown="\"Autodrive\"" w137 {
              tunnel: w135 -> [w153 w218 w229 w246 w265 w281 w296 w312 w328 w344 _ w368 w390 w405 _ _ _ _]
              tunnel: w131 -> [_ w221 w235 w250 w274 w285 w301 w318 w333 w350 w361 w371 w391 w409 w418 w422 w428 w437]
              tunnel: [w150 w220 w234 w251 w273 w286 w300 w317 w332 w349 w360 w372 w392 w408 w418 w421 w428 w438] -> w147
              tunnel: [w156 TLB_MHL_States."Idle" ("Enum") w237 w252 w270 w289 w303 w316 w334 w348 TLB_MHL_States."Shutdown" ("Enum") w374 w393 w407 TLB_MHL_States."Reset" ("Enum") TLB_MHL_States."Shutdown" ("Enum") TLB_MHL_States."Reset" ("Enum") w435] -> w146
              tunnel: w145 -> [w154 _ _ _ _ _ _ _ _ _ _ _ _ _ _ _ _ _]
              tunnel: w144 -> [w155 _ _ _ _ _ _ _ _ _ _ _ _ _ _ _ _ _]
              tunnel: w133 -> [_ _ w232 w249 w268 _ _ _ _ w347 _ w369 w386 w406 _ _ _ _]
              tunnel: w143 -> [_ _ w227 _ _ _ w295 w311 _ _ _ _ _ _ _ _ _ _]
              tunnel: w142 -> [_ _ _ _ _ _ _ _ _ _ _ _ _ _ _ _ _ w432]
              tunnel: w141 -> [_ _ _ _ _ _ _ _ w327 _ _ _ _ _ _ _ _ _]
              tunnel: w140 -> [_ _ _ _ w264 _ _ _ _ _ _ _ _ _ _ _ _ _]
              tunnel: w139 -> [_ _ _ w247 _ w283 _ _ _ w346 _ _ w385 _ _ _ _ _]
              tunnel: [enum16{"OFF", "ON", "BLINK"}."ON" ("GREEN LED State") enum16{"OFF", "ON", "BLINK"}."OFF" ("GREEN LED State") enum16{"OFF", "ON", "BLINK"}."BLINK" ("GREEN LED State") enum16{"OFF", "ON", "BLINK"}."BLINK" ("GREEN LED State") enum16{"OFF", "ON", "BLINK"}."BLINK" ("GREEN LED State") enum16{"OFF", "ON", "BLINK"}."BLINK" ("GREEN LED State") enum16{"OFF", "ON", "BLINK"}."BLINK" ("GREEN LED State") enum16{"OFF", "ON", "BLINK"}."BLINK" ("GREEN LED State") enum16{"OFF", "ON", "BLINK"}."BLINK" ("GREEN LED State") enum16{"OFF", "ON", "BLINK"}."BLINK" ("GREEN LED State") enum16{"OFF", "ON", "BLINK"}."OFF" ("GREEN LED State") enum16{"OFF", "ON", "BLINK"}."BLINK" ("GREEN LED State") enum16{"OFF", "ON", "BLINK"}."BLINK" ("GREEN LED State") enum16{"OFF", "ON", "BLINK"}."BLINK" ("GREEN LED State") _ enum16{"OFF", "ON", "BLINK"}."OFF" ("GREEN LED State") _ _] -> w132
              tunnel: w131 -> [w151 _ _ _ _ _ _ _ _ _ _ _ _ _ _ _ _ _]
              tunnel: w130 -> [_ _ _ _ _ _ _ _ _ _ _ _ _ _ _ _ _ _]
              tunnel: [_ _ _ _ _ _ _ _ _ _ _ _ w383 _ _ _ _ _] -> w127
              frame "Idle", Default {
                # ">>State Logic >>"
                n142 = Dequeue Element(queue=w153, timeout in ms (-1)=w155, error in (no error)=w154) -> (element=w157:T3)  [unwired: 3 out]
                "element" <- w157
                n143 = case shown="\"Start Drive Straight\"" w157 {
                  tunnel: [TLB_MHL_States."Idle" ("Enum") TLB_MHL_States."Idle" ("Enum") TLB_MHL_States."Task 1" ("Enum") TLB_MHL_States."Task 2" ("Enum") TLB_MHL_States."Task 3" ("Enum") TLB_MHL_States."Task 4" ("Enum") TLB_MHL_States."Shutdown" ("Enum") TLB_MHL_States."Wall follow mode" ("Enum") TLB_MHL_States."Acquire image" ("Enum") TLB_MHL_States."Autodrive" ("Enum")] -> w156
                  tunnel: w151 -> [w158 w160 w164 w171 w177 w185 w192 w199 w206 w213]
                  tunnel: [w158 w160 w163 w170 w178 w184 w191 w198 w205 w211] -> w150
                  frame "Start Sequence" {
                    # "This event should never be triggered"
                  }
                  frame "Idle", Default {
                    # ">>Action states Queue Reference >>"
                  }
                  frame "Start Task 1" {
                    # ">>Action states Queue Reference >>"
                    # "Action items"
                    n144 = for {
                      shift-right: [w168] -> w163
                      shift-left: w164 -> [w167]
                      tunnel: string[] ["Hardware reset", "Software reset", "Forward", ""] -> [w166] mode=indexing
                      n145 = Enqueue Element(queue=w167, element=w166) -> (queue out=w168:refnum<queue>)  [unwired: 2 in, 2 out]
                    }
                  }
                  frame "Start Task 2" {
                    # ">>Action states Queue Reference >>"
                    # "Action items"
                    n146 = for {
                      shift-right: [w175] -> w170
                      shift-left: w171 -> [w174]
                      tunnel: string[] ["Hardware reset", "Software reset", ""] -> [w173] mode=indexing
                      n147 = Enqueue Element(queue=w174, element=w173) -> (queue out=w175:refnum<queue>)  [unwired: 2 in, 2 out]
                    }
                  }
                  frame "Start Task 3" {
                    # ">>Action states Queue Reference >>"
                    n148 = for {
                      shift-right: [w182] -> w178
                      shift-left: w177 -> [w181]
                      tunnel: string[] ["Hardware reset", "Software reset", ""] -> [w180] mode=indexing
                      n149 = Enqueue Element(queue=w181, element=w180) -> (queue out=w182:refnum<queue>)  [unwired: 2 in, 2 out]
                    }
                  }
                  frame "Start Task 4" {
                    # ">>Action states Queue Reference >>"
                    # "Action items"
                    n150 = for {
                      shift-right: [w189] -> w184
                      shift-left: w185 -> [w188]
                      tunnel: string[] ["Hardware reset", "Software reset", ""] -> [w187] mode=indexing
                      n151 = Enqueue Element(queue=w188, element=w187) -> (queue out=w189:refnum<queue>)  [unwired: 2 in, 2 out]
                    }
                  }
                  frame "Exit" {
                    # ">>Action states Queue Reference >>"
                    # "Action items"
                    n152 = for {
                      shift-right: [w196] -> w191
                      shift-left: w192 -> [w195]
                      tunnel: string[] ["Hardware reset", "Software reset", "Motor Control", "Pre-Exit", "Exit"] -> [w194] mode=indexing
                      n153 = Enqueue Element(queue=w195, element=w194) -> (queue out=w196:refnum<queue>)  [unwired: 2 in, 2 out]
                    }
                  }
                  frame "Wall follow mode" {
                    # ">>Action states Queue Reference >>"
                    # "Action items"
                    n154 = for {
                      shift-right: [w203] -> w198
                      shift-left: w199 -> [w202]
                      tunnel: string[] ["Hardware reset", "Software reset", ""] -> [w201] mode=indexing
                      n155 = Enqueue Element(queue=w202, element=w201) -> (queue out=w203:refnum<queue>)  [unwired: 2 in, 2 out]
                    }
                  }
                  frame "Camera vision" {
                    # ">>Action states Queue Reference >>"
                    # "Action items"
                    n156 = for {
                      shift-right: [w210] -> w205
                      shift-left: w206 -> [w209]
                      tunnel: string[] ["Hardware reset", "Software reset", "Cam Init", "Cam Acq"] -> [w208] mode=indexing
                      n157 = Enqueue Element(queue=w209, element=w208) -> (queue out=w210:refnum<queue>)  [unwired: 2 in, 2 out]
                    }
                  }
                  frame "Start Drive Straight" {
                    # ">>Action states Queue Reference >>"
                    # "Action items"
                    n158 = for {
                      shift-right: [w217] -> w211
                      shift-left: w213 -> [w216]
                      tunnel: string[] ["Hardware reset", "Software reset", "Forward", ""] -> [w215] mode=indexing
                      n159 = Enqueue Element(queue=w216, element=w215) -> (queue out=w217:refnum<queue>)  [unwired: 2 in, 2 out]
                    }
                  }
                }
              }
              frame "Startup" {
                # ">>State Logic >>"
                n160 = Flush Queue(queue=w218) -> ()  [unwired: 1 in, 3 out]
                n161 = for {
                  shift-right: [w225] -> w220
                  shift-left: w221 -> [w226]
                  tunnel: string[] ["Init", "NavX Calibrate", "Software reset", "Hardware reset", "Motor Control"] -> [w224] mode=indexing
                  n162 = Enqueue Element(queue=w226, element=w224) -> (queue out=w225:refnum<queue>)  [unwired: 2 in, 2 out]
                }
              }
              frame "Task 1" {
                # ">>State Logic >>"
                n163 = Greater Or Equal?(x=w227, y=1.0) -> (x >= y?=w230:bool)
                n164 = Or(x=w232, y=w230) -> (x .or. y?=w233:bool)
                n165 = case shown="True" w233 {
                  tunnel: [string[] ["Forward", "Motor Control", ""] string[] ["Software reset", "Hardware reset", "Motor Control"]] -> w236
                  frame False {
                  }
                  frame True {
                  }
                }
                n166 = Flush Queue(queue=w229) -> ()  [unwired: 1 in, 3 out]
                n167 = Select(t=TLB_MHL_States."Idle" ("Enum"), s=w233, f=TLB_MHL_States."Task 1" ("Enum")) -> (s? t:f=w237:T4)
                n168 = for {
                  shift-right: [w243] -> w234
                  shift-left: w235 -> [w244]
                  tunnel: w236 -> [w242] mode=indexing
                  n169 = Enqueue Element(queue=w244, element=w242) -> (queue out=w243:refnum<queue>)  [unwired: 2 in, 2 out]
                }
              }
              frame "Task 2" {
                # ">>State Logic >>"
                n170 = Flush Queue(queue=w246) -> ()  [unwired: 1 in, 3 out]
                n171 = case shown="True" w249 {
                  tunnel: [w256 string[] ["Hardware reset", "Software reset", "Motor control"]] -> w248
                  tunnel: w247 -> [w255 _]
                  frame False {
                    n172 = case shown="False" w255 {
                      tunnel: [string[] ["Stop", "Ultrasonic read", "Motor Control"] string[] ["Reverse", "Ultrasonic read", "Motor control"]] -> w256
                      frame False {
                      }
                      frame True {
                      }
                    }
                  }
                  frame True {
                  }
                }
                n173 = Select(t=TLB_MHL_States."Idle" ("Enum"), s=w249, f=TLB_MHL_States."Task 2" ("Enum")) -> (s? t:f=w252:T4)
                n174 = for {
                  shift-right: [w261] -> w251
                  shift-left: w250 -> [w262]
                  tunnel: w248 -> [w260] mode=indexing
                  n175 = Enqueue Element(queue=w262, element=w260) -> (queue out=w261:refnum<queue>)  [unwired: 2 in, 2 out]
                }
              }
              frame "Task 3" {
                n176 = Greater Or Equal?(x=w264, y=360.0) -> (x >= y?=w267:bool)
                n177 = Flush Queue(queue=w265) -> ()  [unwired: 1 in, 3 out]
                n178 = Or(x=w267, y=w268) -> (x .or. y?=w269:bool)
                n179 = case shown="False" w269 {
                  tunnel: [string[] ["Rotate CW", "Motor Control"] string[] ["Software reset", "Hardware reset", "Motor Control"]] -> w275
                  frame False {
                  }
                  frame True {
                  }
                }
                n180 = for {
                  shift-right: [w277] -> w273
                  shift-left: w274 -> [w278]
                  tunnel: w275 -> [w276] mode=indexing
                  n181 = Enqueue Element(queue=w278, element=w276) -> (queue out=w277:refnum<queue>)  [unwired: 2 in, 2 out]
                }
                n182 = Select(t=TLB_MHL_States."Idle" ("Enum"), s=w269, f=TLB_MHL_States."Task 3" ("Enum")) -> (s? t:f=w270:T4)
              }
              frame "Task 4" {
                n183 = Flush Queue(queue=w281) -> ()  [unwired: 1 in, 3 out]
                n184 = case shown="True" w283 {
                  tunnel: [string[] ["Forward", "Ultrasonic read", "Motor Control"] string[] ["Stop", "Hardware reset", "Software reset", "Motor Control"]] -> w284
                  frame False {
                  }
                  frame True {
                  }
                }
                n185 = for {
                  shift-right: [w293] -> w286
                  shift-left: w285 -> [w294]
                  tunnel: w284 -> [w292] mode=indexing
                  n186 = Enqueue Element(queue=w294, element=w292) -> (queue out=w293:refnum<queue>)  [unwired: 2 in, 2 out]
                }
                n187 = Select(t=TLB_MHL_States."Task 4a" ("Enum"), s=w283, f=TLB_MHL_States."Task 4" ("Enum")) -> (s? t:f=w289:T4)
              }
              frame "Task 4a" {
                n188 = Greater Or Equal?(x=w295, y=0.5) -> (x >= y?=w299:bool)
                n189 = Flush Queue(queue=w296) -> ()  [unwired: 1 in, 3 out]
                n190 = case shown="True" w299 {
                  tunnel: [string[] ["Right", "Motor Control"] string[] ["Stop", "Hardware reset", "Software reset", "Motor Control"]] -> w302
                  frame False {
                  }
                  frame True {
                  }
                }
                n191 = for {
                  shift-right: [w309] -> w300
                  shift-left: w301 -> [w310]
                  tunnel: w302 -> [w308] mode=indexing
                  n192 = Enqueue Element(queue=w310, element=w308) -> (queue out=w309:refnum<queue>)  [unwired: 2 in, 2 out]
                }
                n193 = Select(t=TLB_MHL_States."Task 4b" ("Enum"), s=w299, f=TLB_MHL_States."Task 4a" ("Enum")) -> (s? t:f=w303:T4)
              }
              frame "Task 4b" {
                n194 = Flush Queue(queue=w312) -> ()  [unwired: 1 in, 3 out]
                n195 = Greater Or Equal?(x=w311, y=0.75) -> (x >= y?=w314:bool)
                n196 = case shown="False" w314 {
                  tunnel: [string[] ["Forward", "Motor control"] string[] ["Stop", "Hardware reset", "Software reset"]] -> w319
                  frame False {
                  }
                  frame True {
                  }
                }
                n197 = for {
                  shift-right: [w325] -> w317
                  shift-left: w318 -> [w326]
                  tunnel: w319 -> [w324] mode=indexing
                  n198 = Enqueue Element(queue=w326, element=w324) -> (queue out=w325:refnum<queue>)  [unwired: 2 in, 2 out]
                }
                n199 = Select(t=TLB_MHL_States."Task 4c" ("Enum"), s=w314, f=TLB_MHL_States."Task 4b" ("Enum")) -> (s? t:f=w316:T4)
              }
              frame "Task 4c" {
                n200 = Flush Queue(queue=w328) -> ()  [unwired: 1 in, 3 out]
                n201 = Less Or Equal?(x=w327, y=-0.65) -> (x <= y?=w330:bool)
                n202 = case shown="False" w330 {
                  tunnel: [string[] ["Left", "Motor Control"] string[] ["Stop", "Hardware reset", "Software reset", "Motor Control"]] -> w335
                  frame False {
                  }
                  frame True {
                  }
                }
                n203 = for {
                  shift-right: [w341] -> w332
                  shift-left: w333 -> [w342]
                  tunnel: w335 -> [w340] mode=indexing
                  n204 = Enqueue Element(queue=w342, element=w340) -> (queue out=w341:refnum<queue>)  [unwired: 2 in, 2 out]
                }
                n205 = Select(t=TLB_MHL_States."Task 4d" ("Enum"), s=w330, f=TLB_MHL_States."Task 4c" ("Enum")) -> (s? t:f=w334:T4)
              }
              frame "Task 4d" {
                n206 = Flush Queue(queue=w344) -> ()  [unwired: 1 in, 3 out]
                n207 = Or(x=w347, y=w346) -> (x .or. y?=w345:bool)
                n208 = case shown="True" w345 {
                  tunnel: [string[] ["Forward", "Ultrasonic Read", "Motor Control"] string[] ["Stop", "Hardware reset", "Software reset", "Motor Control"]] -> w351
                  frame False {
                  }
                  frame True {
                  }
                }
                n209 = for {
                  shift-right: [w357] -> w349
                  shift-left: w350 -> [w358]
                  tunnel: w351 -> [w356] mode=indexing
                  n210 = Enqueue Element(queue=w358, element=w356) -> (queue out=w357:refnum<queue>)  [unwired: 2 in, 2 out]
                }
                n211 = Select(t=TLB_MHL_States."Idle" ("Enum"), s=w345, f=TLB_MHL_States."Task 4d" ("Enum")) -> (s? t:f=w348:T4)
              }
              frame "Reset" {
                n212 = for {
                  shift-right: [w365] -> w360
                  shift-left: w361 -> [w366]
                  tunnel: string[] ["Software reset", "Hardware reset", "Motor Control"] -> [w364] mode=indexing
                  n213 = Enqueue Element(queue=w366, element=w364) -> (queue out=w365:refnum<queue>)  [unwired: 2 in, 2 out]
                }
              }
              frame "Wall follow mode" {
                n214 = Flush Queue(queue=w368) -> ()  [unwired: 1 in, 3 out]
                n215 = case shown="False" w369 {
                  tunnel: [string[] ["IR Sensor Read", "Calculate", "Forward", "Motor Control"] string[] ["Hardware reset", "Software reset", "Motor Control"]] -> w370
                  frame False {
                  }
                  frame True {
                  }
                }
                n216 = for {
                  shift-right: [w379] -> w372
                  shift-left: w371 -> [w380]
                  tunnel: w370 -> [w378] mode=indexing
                  n217 = Enqueue Element(queue=w380, element=w378) -> (queue out=w379:refnum<queue>)  [unwired: 2 in, 2 out]
                }
                n218 = Select(t=TLB_MHL_States."Idle" ("Enum"), s=w369, f=TLB_MHL_States."Wall follow mode" ("Enum")) -> (s? t:f=w374:T4)
              }
              frame "Autodrive" {
                # ">>>Return to idle event>>>"
                n219 = Flush Queue(queue=w390) -> ()  [unwired: 1 in, 3 out]
                n220 = Boolean To (0,1)(Boolean=w386) -> (0, 1=w388:i16)
                n221 = Boolean To (0,1)(Boolean=w385) -> (0, 1=w387:i16)
                n222 = formula code="if (detect == 0 && stop == 0)\nout = 0;\n\nelse if (detect == 1 && stop == 0)\nout = 1;\n\nelse if (detect == 0 && stop == 1)\nout = 2;\n\nelse if (detect == 1 && stop == 1)\nout = 2;"("stop"=w388, "detect"=w387) -> ("out"=w384:dbl)
                n223 = To Byte Integer(number=w384) -> (8bit integer=w383:i8)
                n224 = case shown="0, Default" w383 {
                  tunnel: [string[] ["Forward", "Ultrasonic read"] string[] ["Hardware reset", "Software reset", "Rotate Clockwise", ""] string[] ["Hardware reset", "Software reset", "Motor Control", ""]] -> w381
                  frame 0, Default {
                  }
                  frame 1 {
                  }
                  frame 2 {
                  }
                }
                n225 = for {
                  shift-right: [w402] -> w392
                  shift-left: w391 -> [w403]
                  tunnel: w381 -> [w401] mode=indexing
                  n226 = Enqueue Element(queue=w403, element=w401) -> (queue out=w402:refnum<queue>)  [unwired: 2 in, 2 out]
                }
                n227 = case shown="0, Default" w383 {
                  tunnel: [TLB_MHL_States."Autodrive" ("Enum") TLB_MHL_States."Autodrive a" ("Enum") TLB_MHL_States."Idle" ("Enum")] -> w382
                  frame 0, Default {
                  }
                  frame 1 {
                  }
                  frame 2 {
                  }
                }
                n228 = Select(t=w382, s=w386, f=TLB_MHL_States."Autodrive" ("Enum")) -> (s? t:f=w393:T4)
              }
              frame "Acquire image" {
                n229 = Flush Queue(queue=w405) -> ()  [unwired: 1 in, 3 out]
                n230 = case shown="True" w406 {
                  tunnel: [string[] ["Cam Acq"] string[] ["Hardware reset", "Software reset", "Cam Exit", ""]] -> w410
                  frame False {
                  }
                  frame True {
                  }
                }
                n231 = for {
                  shift-right: [w416] -> w408
                  shift-left: w409 -> [w417]
                  tunnel: w410 -> [w415] mode=indexing
                  n232 = Enqueue Element(queue=w417, element=w415) -> (queue out=w416:refnum<queue>)  [unwired: 2 in, 2 out]
                }
                n233 = Select(t=TLB_MHL_States."Idle" ("Enum"), s=w406, f=TLB_MHL_States."Acquire image" ("Enum")) -> (s? t:f=w407:T4)
              }
              frame "Processing" {
              }
              frame "Shutdown" {
                # ">>State Logic >>"
                n234 = for {
                  shift-right: [w426] -> w421
                  shift-left: w422 -> [w427]
                  tunnel: string[] ["Software reset", "Hardware reset", "Motor Control", "Cam Exit", "Pre-Exit", "Exit"] -> [w425] mode=indexing
                  n235 = Enqueue Element(queue=w427, element=w425) -> (queue out=w426:refnum<queue>)  [unwired: 2 in, 2 out]
                }
              }
              frame "None" {
              }
              frame "Autodrive a" {
                n236 = Greater Or Equal?(x=w432, y=1.2) -> (x >= y?=w430:bool)
                n237 = case shown="False" w430 {
                  tunnel: [string[] ["Rotate CW", "", ""] string[] ["Stop", "Hardware reset", "Software reset", ""]] -> w436
                  frame False {
                  }
                  frame True {
                  }
                }
                n238 = for {
                  shift-right: [w442] -> w438
                  shift-left: w437 -> [w443]
                  tunnel: w436 -> [w441] mode=indexing
                  n239 = Enqueue Element(queue=w443, element=w441) -> (queue out=w442:refnum<queue>)  [unwired: 2 in, 2 out]
                }
                n240 = Select(t=TLB_MHL_States."Autodrive" ("Enum"), s=w430, f=TLB_MHL_States."Autodrive a" ("Enum")) -> (s? t:f=w435:T4)
              }
            }
            "Decision" <- w127
          }
        }
        n241 = local write "GREEN LED State"(w101) -> ()
      }
      n242 = call <vilib>:"NavX Close.vi"("NavX Info In"=w28) -> ()  [unwired: 10 in, 1 out]
      n243 = while {
        shift-right: [w62] -> _
        shift-left: _ -> [w63]
        shift-right: [w61] -> _
        shift-left: _ -> [w60]
        stop <- w69 stop-if-true
        (unwired) TRUE
        # "LED Blinker Loop"
        n244 = case shown="\"BLINK\"" "GREEN LED State" {
          tunnel: [FALSE TRUE w77] -> w65
          tunnel: w63 -> [_ _ w77]
          tunnel: [_ _ w78] -> w62
          frame "OFF", Default {
          }
          frame "ON" {
          }
          frame "BLINK" {
            n245 = Not(x=w77) -> (.not. x?=w78:bool)
          }
        }
        n246 = case shown="\"OFF\", Default" "RED LED State" {
          tunnel: [FALSE TRUE w73] -> w64
          tunnel: [_ _ w74] -> w61
          tunnel: w60 -> [_ _ w73]
          frame "OFF", Default {
          }
          frame "ON" {
          }
          frame "BLINK" {
            n247 = Not(x=w73) -> (.not. x?=w74:bool)
          }
        }
        n248 = local write "Green LED"(w65) -> ()
        n249 = local write "Red LED"(w64) -> ()
        n250 = call "FGV Stop.vi"("Init/Read/Write State"=States_for_Action_Engine."Read") -> ("Output node"=w69:bool)  [unwired: 2 in, 1 out]
        n251 = Wait (ms)(milliseconds to wait=u32 500) -> ()  [unwired: 1 out]
      }
      n252 = call <vilib>:"DIO Close.vi"("DIO Info In"=w3) -> ()  [unwired: 10 in, 1 out]
      n253 = call <vilib>:"DIO Close.vi"("error in (no error)"=w20, "DIO Info In"=w26) -> ()  [unwired: 9 in, 1 out]
      n254 = call <vilib>:"DIO Close.vi"("error in (no error)"=w18, "DIO Info In"=w22) -> ()  [unwired: 9 in, 1 out]
      n255 = call <vilib>:"DIO Close.vi"("error in (no error)"=w8, "DIO Info In"=w13) -> ()  [unwired: 9 in, 1 out]
      n256 = call <vilib>:"DIO Close.vi"("error in (no error)"=w6, "DIO Info In"=w12) -> ()  [unwired: 9 in, 1 out]
      n257 = Merge Errors "Merge Errors"(w53, w52) -> (w34:errorcluster)
      n258 = Merge Errors(w38, w34) -> (w29:errorcluster)
      n259 = Destroy User Event(user event=w56, error in=w29) -> ()  [unwired: 1 out]
      n260 = Destroy User Event(user event=w57, error in=w29) -> ()  [unwired: 1 out]
      n261 = Unregister For Events(event registration refnum=w48, error in=w29) -> ()  [unwired: 1 out]
      n262 = Release Queue(queue=w31, error in (no error)=w29) -> (error out=→"error out":errorcluster)  [unwired: 1 in, 2 out]
      n263 = Release Queue(queue=w47, error in (no error)=w29) -> ()  [unwired: 1 in, 3 out]
    }
    frame #2 {
      (unwired) T14."INIT" ("States")
      n264 = call "New motor Control integrated remodeled state based.vi"() -> ()  [unwired: 3 in, 2 out]
    }
    frame #3 {
    }
  }
